vi "Home.vi"(8 "error in (no error)":errorcluster, 10 "Enum":enum16{"No", "Home", "Anneal"}(ring), 11 "TCP Network Connection in":refnum<k5>) -> (0 "error out":errorcluster, 2 "Command Status":bool, 3 "TCP Network Connection out":refnum<k5>)   [LabVIEW 2019]
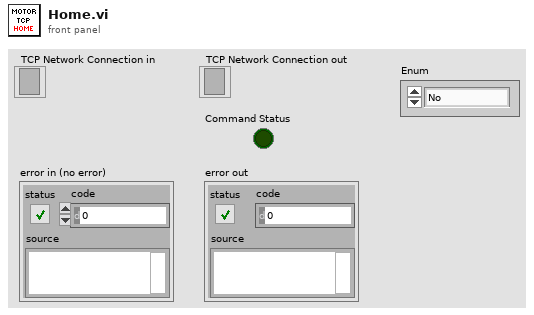
[diagram p1: front panel]
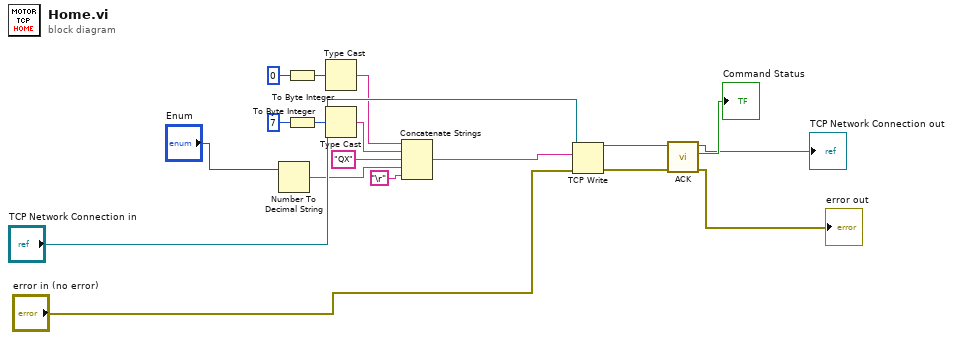
[diagram p0: block diagram]
diagram:
  n1 = Number To Decimal String(number="Enum") -> (decimal integer string=w3:string)  [unwired: 1 in]
  n2 = To Byte Integer(number=i8 0) -> (8bit integer=w8:i8)
  n3 = To Byte Integer(number=i8 7) -> (8bit integer=w5:i8)
  n4 = Type Cast(x=w8) -> (*(type *) &x=w7:string)  [unwired: 1 in]
  n5 = Type Cast(x=w5) -> (*(type *) &x=w6:string)  [unwired: 1 in]
  n6 = Concatenate Strings(w7, w6, "QX" ("string"), w3, "\r") -> (w11:string)
  n7 = TCP Write(connection ID="TCP Network Connection in", data in=w11, error in (no error)="error in (no error)") -> (connection ID out=w14:refnum<k5>, error out=w15:errorcluster)  [unwired: 1 in, 1 out]
  n8 = call "ACK.vi"("error in (no error)"=w15, "TCP Network Connection in"=w14) -> ("error out"=→"error out":errorcluster, "Command Status"=→"Command Status":bool, "TCP Network Connection out"=→"TCP Network Connection out":refnum<k5>)  [unwired: 7 in]
